vi "Global variables.vi"() -> ()   [LabVIEW 2020]
panel:
  in  "Proton's mass":dbl
  in  "Energy from modules":dbl
  in  "Speed of light":dbl
  in  "Starting energy":dbl=1e-06
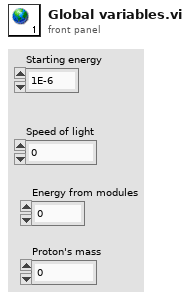
[diagram p1: front panel]
diagram:
